vi "stat 32 to stat 64.vi"(11 "stat 32":T12) -> (3 "stat 64":T1)   [LabVIEW 2013, in "Linux RT IPC.lvlib" / "C.lvlib"]
uses:
  C.lvlib
  Controls/C Types/stat_32.ctl
  Controls/C Types/dev_t.ctl
  Controls/C Types/ino_t_32.ctl
  Controls/C Types/mode_t.ctl
  Controls/C Types/nlink_t_32.ctl
  Controls/C Types/uid_t.ctl
  Controls/C Types/gid_t.ctl
  Controls/C Types/off_t_32.ctl
  Controls/C Types/blksize_t_32.ctl
  Controls/C Types/blkcnt_t_32.ctl
  Controls/C Types/time_t_32.ctl
  Controls/C Types/stat_64.ctl
  Controls/C Types/ino_t_64.ctl
  Controls/C Types/nlink_t_64.ctl
  Controls/C Types/off_t_64.ctl
  Controls/C Types/blksize_t_64.ctl
  Controls/C Types/blkcnt_t_64.ctl
  Controls/C Types/time_t_64.ctl
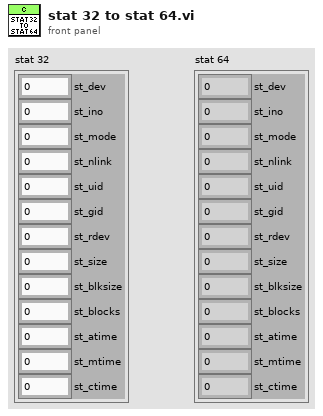
[diagram p1: front panel]
types:
  T1 = typedef "Linux RT IPC.lvlib/C.lvlib/stat_64.ctl" = cluster{"st_dev":T2, "st_ino":T3, "st_mode":T4, "st_nlink":T5, "st_uid":T6, "st_gid":T7, "st_rdev":T2, "st_size":T8, "st_blksize":T9, "st_blocks":T10, "st_atime":T11, "st_mtime":T11, "st_ctime":T11}
  T2 = typedef "Linux RT IPC.lvlib/C.lvlib/dev_t.ctl" = u64
  T3 = typedef "Linux RT IPC.lvlib/C.lvlib/ino_t_64.ctl" = u64
  T4 = typedef "Linux RT IPC.lvlib/C.lvlib/mode_t.ctl" = u32
  T5 = typedef "Linux RT IPC.lvlib/C.lvlib/nlink_t_64.ctl" = u64
  T6 = typedef "Linux RT IPC.lvlib/C.lvlib/uid_t.ctl" = u32
  T7 = typedef "Linux RT IPC.lvlib/C.lvlib/gid_t.ctl" = u32
  T8 = typedef "Linux RT IPC.lvlib/C.lvlib/off_t_64.ctl" = u64
  T9 = typedef "Linux RT IPC.lvlib/C.lvlib/blksize_t_64.ctl" = u64
  T10 = typedef "Linux RT IPC.lvlib/C.lvlib/blkcnt_t_64.ctl" = u64
  T11 = typedef "Linux RT IPC.lvlib/C.lvlib/time_t_64.ctl" = u64
  T12 = typedef "Linux RT IPC.lvlib/C.lvlib/stat_32.ctl" = cluster{"st_dev":T2, "st_ino":T13, "st_mode":T4, "st_nlink":T14, "st_uid":T6, "st_gid":T7, "st_rdev":T2, "st_size":T15, "st_blksize":T16, "st_blocks":T17, "st_atime":T18, "st_mtime":T18, "st_ctime":T18}
  T13 = typedef "Linux RT IPC.lvlib/C.lvlib/ino_t_32.ctl" = u32
  T14 = typedef "Linux RT IPC.lvlib/C.lvlib/nlink_t_32.ctl" = u32
  T15 = typedef "Linux RT IPC.lvlib/C.lvlib/off_t_32.ctl" = u32
  T16 = typedef "Linux RT IPC.lvlib/C.lvlib/blksize_t_32.ctl" = u32
  T17 = typedef "Linux RT IPC.lvlib/C.lvlib/blkcnt_t_32.ctl" = u32
  T18 = typedef "Linux RT IPC.lvlib/C.lvlib/time_t_32.ctl" = u32
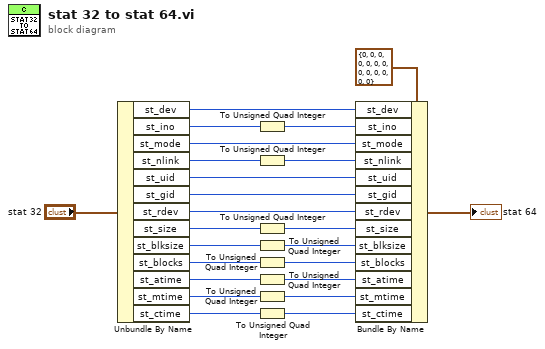
[diagram p0: block diagram]
diagram:
  n1 = Unbundle By Name("stat 32") -> ("st_dev"=w21:T2, "st_ino"=w20:T13, "st_mode"=w19:T4, "st_nlink"=w18:T14, "st_uid"=w17:T6, "st_gid"=w16:T7, "st_rdev"=w15:T2, "st_size"=w14:T15, "st_blksize"=w13:T16, "st_blocks"=w12:T17, "st_atime"=w11:T18, "st_mtime"=w10:T18, "st_ctime"=w9:T18)
  n2 = To Unsigned Quad Integer(1:w20) -> (0:w8:u64)
  n3 = To Unsigned Quad Integer(1:w18) -> (0:w7:u64)
  n4 = To Unsigned Quad Integer(1:w14) -> (0:w6:u64)
  n5 = To Unsigned Quad Integer(1:w13) -> (0:w5:u64)
  n6 = To Unsigned Quad Integer(1:w12) -> (0:w4:u64)
  n7 = To Unsigned Quad Integer(1:w11) -> (0:w3:u64)
  n8 = To Unsigned Quad Integer(1:w10) -> (0:w2:u64)
  n9 = To Unsigned Quad Integer(1:w9) -> (0:w1:u64)
  n10 = Bundle By Name(cluster=T1 {"st_dev"=0, "st_ino"=0, "st_mode"=0, "st_nlink"=0, "st_uid"=0, "st_gid"=0, "st_rdev"=0, "st_size"=0, "st_blksize"=0, "st_blocks"=0, "st_atime"=0, "st_mtime"=0, "st_ctime"=0} ("stat"), "st_dev"=w21, "st_ino"=w8, "st_mode"=w19, "st_nlink"=w7, "st_uid"=w17, "st_gid"=w16, "st_rdev"=w15, "st_size"=w6, "st_blksize"=w5, "st_blocks"=w4, "st_atime"=w3, "st_mtime"=w2, "st_ctime"=w1) -> (→"stat 64":T1)
